vi "Sent_CAN.vi"(6 "帧长度":u8, 7 "帧类型":u8, 8 "error in (no error)":errorcluster, 9 "帧数据":T1, 10 "帧格式":u8, 11 "ID":u32) -> (0 "error out":errorcluster)   [LabVIEW 2020, in "ZLG_CAN.lvlib"]
doc: "_____\nCreated using Delacor QMH Event Scripter 4.1.0.80."
uses:
  ZLG_CAN.lvlib
  CAN_Frame.ctl
  Sent_CAN Argument--cluster.ctl
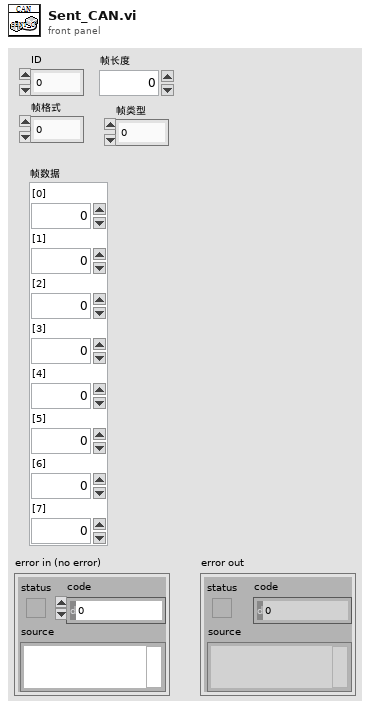
[diagram p1: front panel]
types:
  T1 = typedef "ZLG_CAN.lvlib/CAN_Frame.ctl" = cluster{"[0]":u8, "[1]":u8, "[2]":u8, "[3]":u8, "[4]":u8, "[5]":u8, "[6]":u8, "[7]":u8}
  T2 = typedef "ZLG_CAN.lvlib/Sent_CAN Argument--cluster.ctl" = cluster{"ID":u32, "帧类型":u8, "帧格式":u8, "帧长度":u8, "CAN_FRAME":T1}
  T3 = typedef "ZLG_CAN.lvlib/Request Events--cluster.ctl" = cluster{"Stop Module":refnum<user-event>, "Show Panel":refnum<user-event>, "Hide Panel":refnum<user-event>, "Get Module Execution Status":refnum<user-event>, "Show Diagram":refnum<user-event>, "Open_CAN":refnum<user-event>, "Init_CAN":refnum<user-event>, "Start_CAN":refnum<user-event>, "Sent_CAN":refnum<user-event>, "Close_CAN":refnum<user-event>, "Reset_CAN":refnum<user-event>, "Recive_CAN":refnum<user-event>, "Recive_Wait":refnum<user-event>, "Sent_Recive":refnum<user-event>}
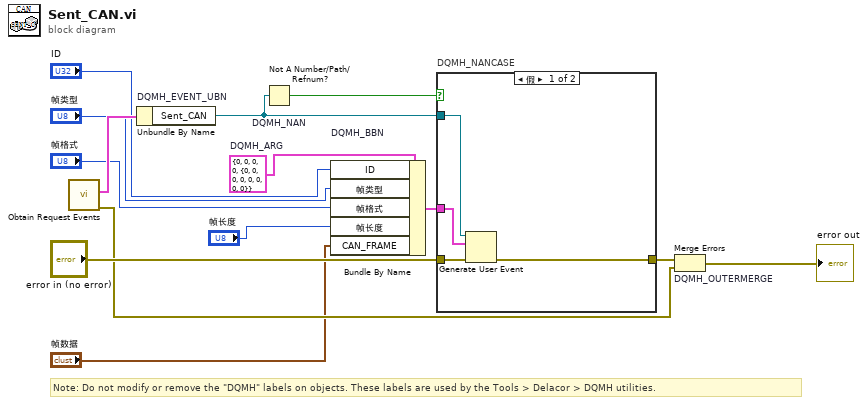
[diagram p0: block diagram]
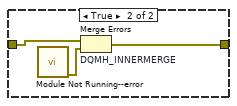
[diagram p2: hidden frame]
diagram:
  w8 = T2 {"ID"=0, "帧类型"=0, "帧格式"=0, "帧长度"=0, "CAN_FRAME"={"[0]"=0, "[1]"=0, "[2]"=0, "[3]"=0, "[4]"=0, "[5]"=0, "[6]"=0, "[7]"=0}}  # DQMH_ARG
  # "Note: Do not modify or remove the \"DQMH\" labels on objects. These labels are used by the Tools > Delacor > DQMH utilities."
  n1 = call "Obtain Request Events.vi"() -> ("error out"=w7:errorcluster, "ZLG_CAN Request Events"=w6:T3)  [unwired: 10 in]
  n2 = Unbundle By Name "DQMH_EVENT_UBN"(w6) -> ("Sent_CAN"=w10:refnum<user-event>)
  n3 = Not A Number/Path/Refnum? "DQMH_NAN"(number/path/refnum=w10) -> (NaN/Path/Refnum?=w11:bool)
  n4 = Bundle By Name "DQMH_BBN"(cluster=w8, "ID"="ID", "帧类型"="帧类型", "帧格式"="帧格式", "帧长度"="帧长度", "CAN_FRAME"="帧数据") -> (w12:T2)
  n5 = case "DQMH_NANCASE" shown="假" w11 {
    tunnel: "error in (no error)" -> [w18 w21]
    tunnel: [w17 w20] -> w9
    tunnel: w10 -> [w16 _]
    tunnel: w12 -> [w15 _]
    frame False {
      n6 = Generate User Event(user event=w16, event data cluster=w15, error in=w18) -> (error out=w17:errorcluster)  [unwired: 1 in, 1 out]
    }
    frame True {
      n7 = call "Module Not Running--error.vi"() -> ("error out"=w19:errorcluster)  [unwired: 11 in]
      n8 = Merge Errors "DQMH_INNERMERGE"(w21, w19) -> (w20:errorcluster)
    }
  }
  n9 = Merge Errors "DQMH_OUTERMERGE"(w9, w7) -> (→"error out":errorcluster)
